vi "Prepare Control.vi"(7 "VolatusAPI":refnum<class "VolatusAPI.lvclass">, 8 "error in (no error)":errorcluster, 11 "ValveControl in":refnum<class "PeriodicControl.lvclass">) -> (0 "error out":errorcluster, 3 "ValveControl out":refnum<class "PeriodicControl.lvclass">)   [LabVIEW 2020, in "VolatusControl.lvlib" / "PeriodicControl.lvclass"]
uses:
  PeriodicControl.lvclass
  Volatus/VolatusAPI/VolatusAPI.lvclass
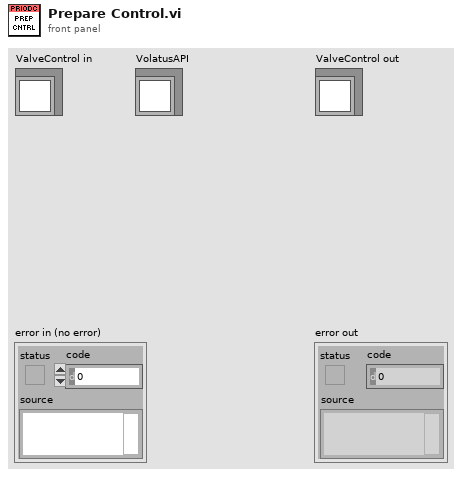
[diagram p1: front panel]
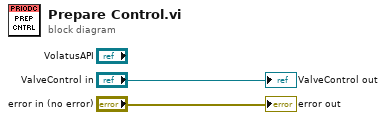
[diagram p0: block diagram]
diagram:
  "error out" <- "error in (no error)"
  "ValveControl out" <- "ValveControl in"
